vi "Read Data.vi"(8 "AI Rate":dbl=10000.0 format="%.2f", 9 "AI Buffer Size (s)":i32=10, 10 "AI Block Size":i32=5000, 11 "AI task":refnum<k21>[](array[refnum])=["", ""]) -> (1 "Backlog":u8(slide) scale=0.0..100.0, 2 "Input Signals":dbl[][](array[numeric]), 3 "Input Signals":waveform(dbl)[](array[waveform]))   [LabVIEW 2013]
uses:
  <vilib>/DAQmx/read.llb/DAQmx Read (Analog 1D Wfm NChan NSamp).vi
  <vilib>/DAQmx/miscellaneous.llb/DAQmx Fill In Error Info.vi
  <vilib>/DAQmx/read.llb/DAQmx Read (Analog 2D DBL NChan NSamp).vi
  <resource>/objmgr/daqmx.rc
panel:
  out "Waveform Graph":waveform(dbl)[](graph)
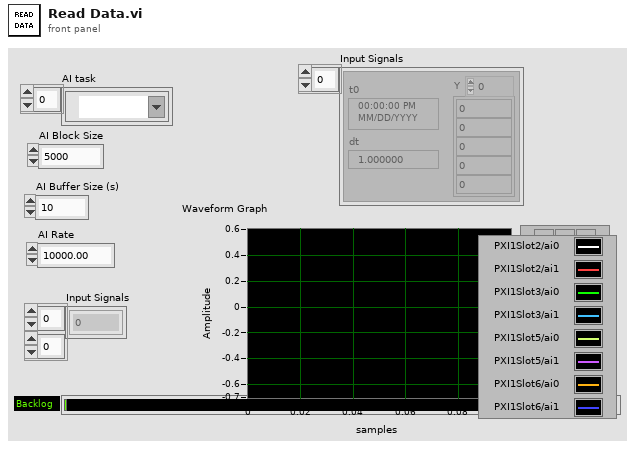
[diagram p1: front panel]
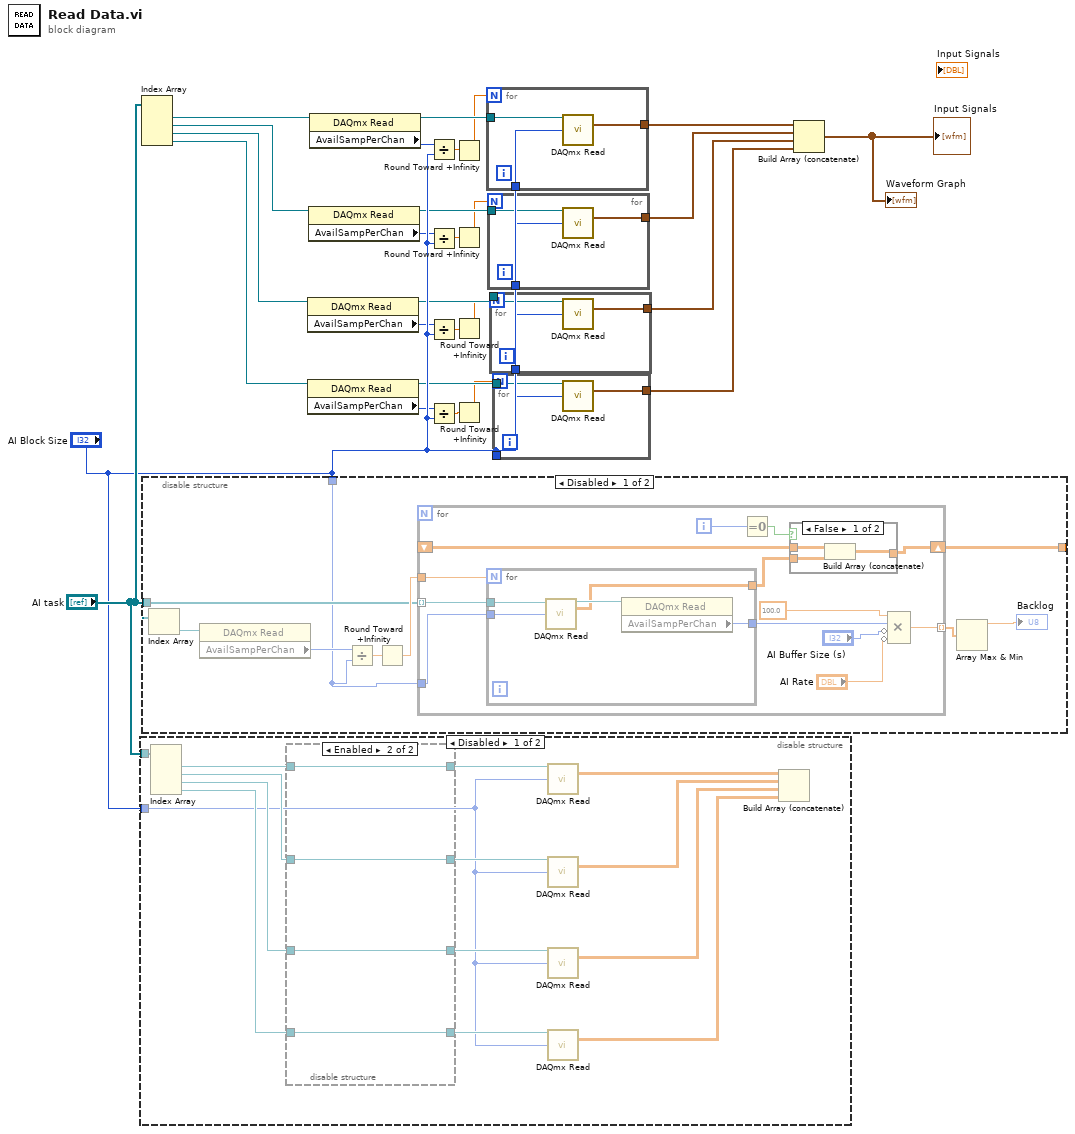
[diagram p0: block diagram]
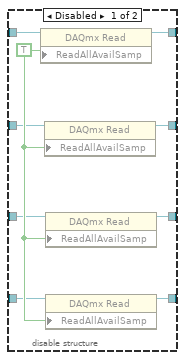
[diagram p2: hidden frame]
diagram:
  n1 = disable-structure shown="Disabled" {
    disable-tunnel: "AI task" -> [w41 _]
    disable-tunnel: "AI Block Size" -> [w28 _]
    frame Disabled {
      n2 = Index Array(array=w41) -> (element #1=w40:refnum<k21>, element #2=w35:refnum<k21>, element #3=w34:refnum<k21>, element #4=w33:refnum<k21>)  [unwired: 4 in]
      n3 = disable-structure shown="Enabled" {
        disable-tunnel: w40 -> [w50 w54]
        disable-tunnel: [w49 w54] -> w39
        disable-tunnel: [w48 w51] -> w38
        disable-tunnel: [w47 w52] -> w37
        disable-tunnel: [w46 w53] -> w36
        disable-tunnel: w35 -> [w44 w53]
        disable-tunnel: w34 -> [w43 w52]
        disable-tunnel: w33 -> [w42 w51]
        frame Disabled {
          w45 = TRUE ("ReadAllAvailSamp")
          n4 = property class="DAQmx Read"(reference=w50, "ReadAllAvailSamp"=w45) -> (reference out=w49:refnum<k21>)  [unwired: 1 in, 1 out]
          n5 = property class="DAQmx Read"(reference=w44, "ReadAllAvailSamp"=w45) -> (reference out=w46:refnum<k21>)  [unwired: 1 in, 1 out]
          n6 = property class="DAQmx Read"(reference=w43, "ReadAllAvailSamp"=w45) -> (reference out=w47:refnum<k21>)  [unwired: 1 in, 1 out]
          n7 = property class="DAQmx Read"(reference=w42, "ReadAllAvailSamp"=w45) -> (reference out=w48:refnum<k21>)  [unwired: 1 in, 1 out]
        }
        frame Enabled {
        }
      }
      n8 = call-poly <vilib>:"DAQmx Read.vi"("task/channels in"=w39, "number of samples per channel"=w28) -> ("data"=w32:dbl[][])  [unwired: 11 in, 2 out]
      n9 = call-poly <vilib>:"DAQmx Read.vi"("task/channels in"=w36, "number of samples per channel"=w28) -> ("data"=w31:dbl[][])  [unwired: 11 in, 2 out]
      n10 = call-poly <vilib>:"DAQmx Read.vi"("task/channels in"=w37, "number of samples per channel"=w28) -> ("data"=w30:dbl[][])  [unwired: 11 in, 2 out]
      n11 = call-poly <vilib>:"DAQmx Read.vi"("task/channels in"=w38, "number of samples per channel"=w28) -> ("data"=w29:dbl[][])  [unwired: 11 in, 2 out]
      n12 = Build Array (concatenate)(w32, w31, w30, w29) -> ()  [unwired: 1 out]
    }
    frame Enabled {
    }
  }
  n13 = Index Array(array="AI task") -> (element #1=w18:refnum<k21>, element #2=w19:refnum<k21>, element #3=w20:refnum<k21>, element #4=w21:refnum<k21>)  [unwired: 4 in]
  n14 = disable-structure shown="Disabled" {
    disable-tunnel: [w57 _] -> _
    disable-tunnel: "AI task" -> [w56 _]
    disable-tunnel: "AI Block Size" -> [w55 _]
    frame Disabled {
      n15 = Index Array(array=w56) -> (element=w61:refnum<k21>)  [unwired: 1 in]
      n16 = property class="DAQmx Read"(reference=w61) -> ("AvailSampPerChan"=w60:u32)  [unwired: 1 in, 2 out]
      n17 = Divide(x=w60, y=w55) -> (x/y=w59:dbl)
      n18 = Round Toward +Infinity(x=w59) -> (ceil(x): smallest int >= x=w58:dbl)
      n19 = for {
        tunnel: w56 -> [w68] mode=indexing
        tunnel: [w74] -> w63 mode=indexing
        shift-right: [w69] -> w57
        shift-left: _ -> [w71]
        tunnel: w58 -> [w67]
        tunnel: w55 -> [w66]
        i -> [w72]
        n20 = for {
          N: w67 -> [_]
          tunnel: [w84] -> w70
          tunnel: [w83] -> w76
          tunnel: w68 -> [w82]
          tunnel: w66 -> [w81]
          n21 = call-poly <vilib>:"DAQmx Read.vi"("task/channels in"=w82, "number of samples per channel"=w81) -> ("task out"=w85:refnum<k21>, "data"=w84:dbl[][])  [unwired: 11 in, 1 out]
          n22 = property class="DAQmx Read"(reference=w85) -> ("AvailSampPerChan"=w83:u32)  [unwired: 1 in, 2 out]
        }
        n23 = Equal To 0?(x=w72) -> (x = 0?=w73:bool)
        n24 = case shown="False" w73 {
          tunnel: w71 -> [w77 _]
          tunnel: w70 -> [w79 w80]
          tunnel: [w78 w80] -> w69
          frame False {
            n25 = Build Array (concatenate)(w77, w79) -> (w78:dbl[][])
          }
          frame True {
          }
        }
        n26 = Compound Arithmetic op=MULTIPLY(100.0 ("value"), w76, invert "AI Buffer Size (s)", invert "AI Rate") -> (w74:dbl)
      }
      n27 = Array Max & Min(array=w63) -> (max value=→"Backlog":dbl)  [unwired: 3 out]
    }
    frame Enabled {
    }
  }
  n28 = property class="DAQmx Read"(reference=w20) -> (reference out=w15:refnum<k21>, "AvailSampPerChan"=w11:u32)  [unwired: 1 in, 1 out]
  n29 = property class="DAQmx Read"(reference=w21) -> (reference out=w14:refnum<k21>, "AvailSampPerChan"=w12:u32)  [unwired: 1 in, 1 out]
  n30 = property class="DAQmx Read"(reference=w19) -> (reference out=w16:refnum<k21>, "AvailSampPerChan"=w10:u32)  [unwired: 1 in, 1 out]
  n31 = property class="DAQmx Read"(reference=w18) -> (reference out=w17:refnum<k21>, "AvailSampPerChan"=w13:u32)  [unwired: 1 in, 1 out]
  n32 = Divide(x=w13, y="AI Block Size") -> (x/y=w9:dbl)
  n33 = Divide(x=w10, y="AI Block Size") -> (x/y=w8:dbl)
  n34 = Divide(x=w11, y="AI Block Size") -> (x/y=w7:dbl)
  n35 = Divide(x=w12, y="AI Block Size") -> (x/y=w6:dbl)
  n36 = Round Toward +Infinity(x=w9) -> (ceil(x): smallest int >= x=w2:dbl)
  n37 = Round Toward +Infinity(x=w8) -> (ceil(x): smallest int >= x=w3:dbl)
  n38 = Round Toward +Infinity(x=w7) -> (ceil(x): smallest int >= x=w4:dbl)
  n39 = Round Toward +Infinity(x=w6) -> (ceil(x): smallest int >= x=w5:dbl)
  n40 = for {
    N: w2 -> [_]
    tunnel: [w88] -> w22
    tunnel: w17 -> [w87]
    tunnel: "AI Block Size" -> [w86]
    n41 = call-poly <vilib>:"DAQmx Read.vi"("task/channels in"=w87, "number of samples per channel"=w86) -> ("data"=w88:waveform(dbl)[])  [unwired: 11 in, 2 out]
  }
  n42 = for {
    N: w3 -> [_]
    tunnel: [w91] -> w23
    tunnel: w16 -> [w90]
    tunnel: "AI Block Size" -> [w89]
    n43 = call-poly <vilib>:"DAQmx Read.vi"("task/channels in"=w90, "number of samples per channel"=w89) -> ("data"=w91:waveform(dbl)[])  [unwired: 11 in, 2 out]
  }
  n44 = for {
    N: w4 -> [_]
    tunnel: [w94] -> w24
    tunnel: w15 -> [w93]
    tunnel: "AI Block Size" -> [w92]
    n45 = call-poly <vilib>:"DAQmx Read.vi"("task/channels in"=w93, "number of samples per channel"=w92) -> ("data"=w94:waveform(dbl)[])  [unwired: 11 in, 2 out]
  }
  n46 = for {
    N: w5 -> [_]
    tunnel: [w97] -> w25
    tunnel: w14 -> [w96]
    tunnel: "AI Block Size" -> [w95]
    n47 = call-poly <vilib>:"DAQmx Read.vi"("task/channels in"=w96, "number of samples per channel"=w95) -> ("data"=w97:waveform(dbl)[])  [unwired: 11 in, 2 out]
  }
  n48 = Build Array (concatenate)(w22, w23, w24, w25) -> (→"Input Signals" →"Waveform Graph":waveform(dbl)[])
